vi "Acquire Waveform.vi"(8 "error in (no error)":errorcluster, 9 "channel list":string, 11 "IVI Refnum in":refnum<k15>) -> (0 "error out":errorcluster, 2 "Measurement Results":T1, 3 "IVI Refnum out":refnum<k15>)   [LabVIEW 2020]
uses:
  Measurement Results.ctl
  IVI Scope Measurement.lvlib
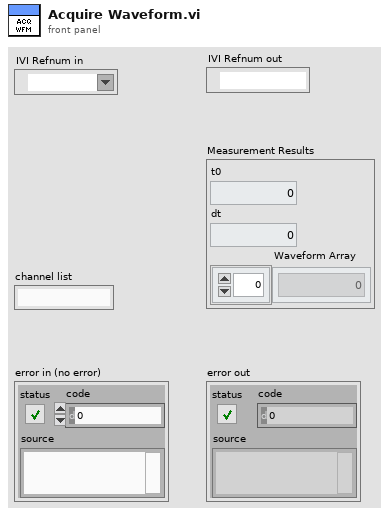
[diagram p1: front panel]
types:
  T1 = typedef "IVI Scope Measurement.lvlib/Measurement Results.ctl" = cluster{"t0":dbl, "dt":dbl, "Waveform Array":dbl[]}
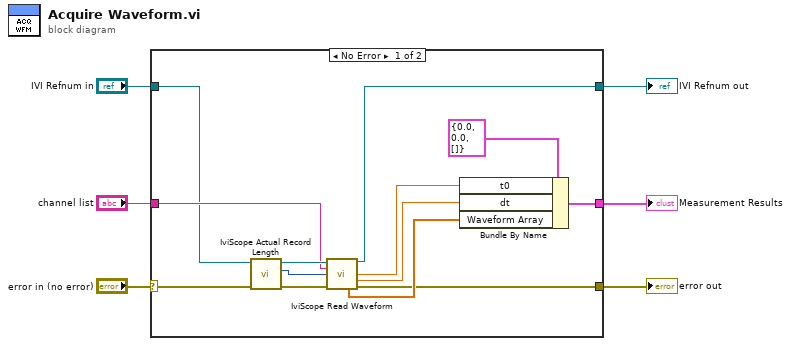
[diagram p0: block diagram]
diagram:
  n1 = case shown="No Error" "error in (no error)" {
    selector: "error in (no error)" -> [w7 w20]
    tunnel: [w12 w20] -> w6
    tunnel: "channel list" -> [w11 _]
    tunnel: "IVI Refnum in" -> [w10 w21]
    tunnel: [w9 _] -> w3
    tunnel: [w8 w21] -> w2
    frame No Error {
      n2 = call <vilib>:"IviScope Actual Record Length.vi"("error in (no error)"=w7, "instrument handle"=w10) -> ("error out"=w14:errorcluster, "actual record length"=w16:i32, "instrument handle out"=w15:refnum<k15>)  [unwired: 7 out]
      n3 = call <vilib>:"IviScope Read Waveform.vi"("instrument handle"=w15, "channel name (\"CHANNEL1\")"=w11, "waveform size (0)"=w16, "error in (no error)"=w14) -> ("instrument handle out"=w8:refnum<k15>, "initial x"=w17:dbl, "x increment"=w18:dbl, "waveform array"=w19:dbl[], "error out"=w12:errorcluster)  [unwired: 2 in, 5 out]
      n4 = Bundle By Name(cluster=T1 {"t0"=0.0, "dt"=0.0, "Waveform Array"=[]} ("Measurement Results"), "t0"=w17, "dt"=w18, "Waveform Array"=w19) -> (w9:T1)
    }
    frame Error {
    }
  }
  "error out" <- w6
  "Measurement Results" <- w3
  "IVI Refnum out" <- w2
